vi "Shared Variable Project Filename and Path--Const.vi"() -> (3 "appended path":path)   [LabVIEW 2017, in "Shared Variables Library.lvlib"]
doc: "The file and path name to the main project, containing the shared variable container library."
uses:
  Shared Variables Library.lvlib
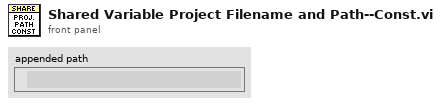
[diagram p1: front panel]
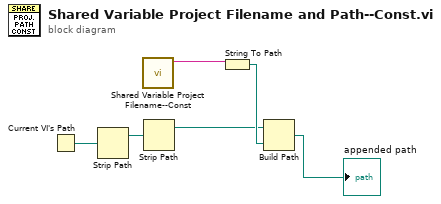
[diagram p0: block diagram]
diagram:
  n1 = Current VI's Path() -> (path=w4:path)
  n2 = Strip Path(path=w4) -> (stripped path=w3:path)  [unwired: 1 out]
  n3 = call "Shared Variable Project Filename--Const.vi"() -> ("Shared Variables Project Filename"=w1:string)  [unwired: 11 in]
  n4 = Strip Path(path=w3) -> (stripped path=w2:path)  [unwired: 1 out]
  n5 = String To Path(string=w1) -> (path=w5:path)
  n6 = Build Path(base path=w2, name or relative path=w5) -> (appended path=→"appended path":path)
